vi "Comandos Inversor.vi"(10 "Argument":string, 11 "Command":T1(ring)) -> (3 "Command":string)   [LabVIEW 2019, in "Inversor.lvlib"]
uses:
  Inversor.lvlib
  <vilib>/regexp/Match Regular Expression.xnode
panel:
  # "Commands Examples\n\nSet Voltage          SV:1000.45\nSet Current          SC:10.02\nSet Frencuency   SF:58.45\nSet Speed             SS:455.05"
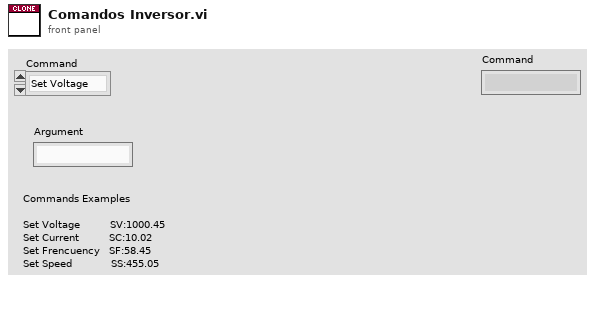
[diagram p1: front panel]
types:
  T1 = enum16{"Set Voltage", "Set Frecuency", "Set Speed", "Set Current"}
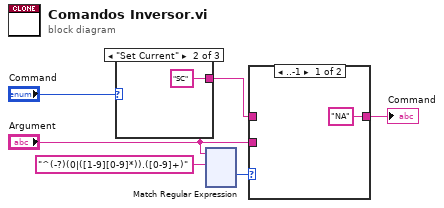
[diagram p0: block diagram]
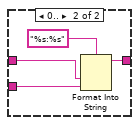
[diagram p2: hidden frame]
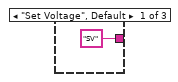
[diagram p3: hidden frame]
diagram:
  n1 = case shown="\"Set Current\"" "Command" {
    tunnel: ["SV" "SC" _] -> w5
    frame "Set Voltage", Default {
    }
    frame "Set Current" {
    }
    frame "Set Frecuency" {
    }
  }
  n2 = xnode "Match Regular Expression"("input string"="Argument", "regular expression"="^(-?)(0|([1-9][0-9]*)).([0-9]+)") -> ("offset past match"=w1:i32)  [unwired: 4 in, 4 out]
  n3 = case shown="..-1" w1 {
    tunnel: w5 -> [_ w13]
    tunnel: "Argument" -> [_ w12]
    tunnel: ["NA" w10] -> w4
    frame ..-1 {
    }
    frame 0.. {
      n4 = Format Into String(format string="%s:%s", w13, w12) -> (resulting string=w10:string)  [unwired: 2 in, 1 out]
    }
  }
  "Command" <- w4
